vi "Read SCPI Error Queue (GPIB).vi"(2 "error in":T1, 3 "GPIB address":string) -> (0 "error out":T1, 1 "messages":string)   [LabVIEW 2024]
doc: "This VI reads the status message from the power meter and determines whether an error has occurred during the previous operations. If an error is detected, the front panel LED (error) will be turned on, and the messages will be displayed."
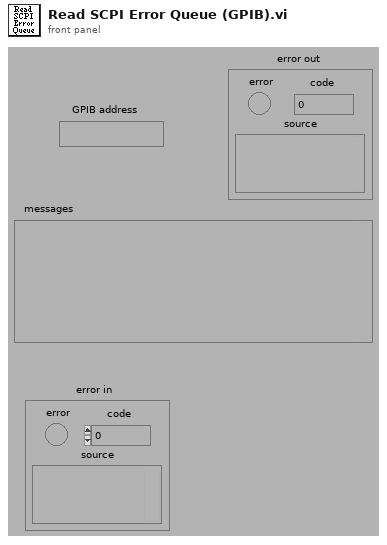
[diagram p1: front panel]
types:
  T1 = cluster{"error":bool, "code":i32, "source":string}
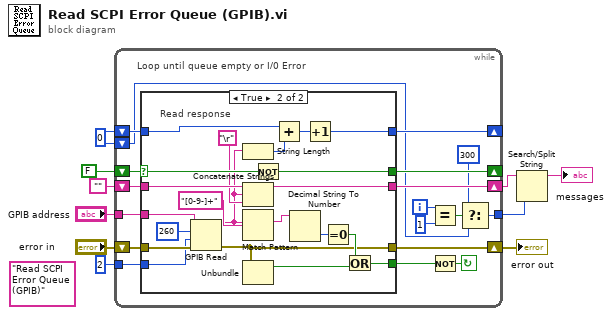
[diagram p0: block diagram]
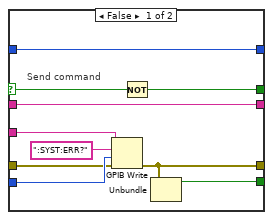
[diagram p2: hidden frame]
diagram:
  w7 = 0
  (unwired) "Read SCPI Error Queue (GPIB)"
  n1 = while {
    shift-right: [w28] -> w6
    shift-left: "" -> [w27]
    shift-right: [w23] -> _
    shift-left: FALSE -> [w24]
    tunnel: "GPIB address" -> [w22]
    shift-right: [w20] -> w1
    shift-left: "error in" -> [w21]
    tunnel: 2 -> [w19]
    shift-right: [w17] -> _
    shift-left: w7 -> [w18]
    shift-left: w7 -> [w16]
    tunnel: [w15] -> w4
    i -> [w14]
    stop <- w25 continue-if-true
    # "Loop until queue empty or I/0 Error"
    n2 = case shown="True" w24 {
      selector: w24 -> [w37 w55]
      tunnel: [w35 w58] -> w26
      tunnel: [w38 w57] -> w28
      tunnel: w27 -> [w38 w56]
      tunnel: [w36 w54] -> w23
      tunnel: w22 -> [w32 w41]
      tunnel: [w33 w43] -> w20
      tunnel: w21 -> [w29 w44]
      tunnel: w19 -> [w30 w40]
      tunnel: w18 -> [w34 w49]
      tunnel: [w34 w47] -> w17
      frame False {
        # "Send command"
        n3 = GPIB Write(0:w32, 1:":SYST:ERR?", 2:w30, 3:w29) -> (6:w33:errorcluster)  [unwired: 1 in, 1 out]
        n4 = Not(x=w37) -> (.not. x?=w36:bool)
        n5 = Unbundle(w33) -> ("status"=w35:bool)  [unwired: 2 out]
      }
      frame True {
        # "Read response"
        n6 = GPIB Read(0:w41, 1:260, 2:w40, 3:w44) -> (5:w42:string, 7:w43:errorcluster)  [unwired: 1 in, 1 out]
        n7 = String Length(string=w42) -> (length=w50:i32)
        n8 = Concatenate Strings(w56, w42, "\r") -> (w57:string)
        n9 = Match Pattern(string=w42, regular expression="[0-9-]+") -> (match substring=w45:string)  [unwired: 1 in, 3 out]
        n10 = Unbundle(w43) -> ("status"=w51:bool)  [unwired: 2 out]
        n11 = Not(x=w55) -> (.not. x?=w54:bool)
        n12 = Add(x=w49, y=w50) -> (x+y=w48:i32)
        n13 = Decimal String To Number(string=w45) -> (number=w59:i32)  [unwired: 2 in, 1 out]
        n14 = Increment(x=w48) -> (x+1=w47:i32)
        n15 = Equal To 0?(x=w59) -> (x = 0?=w53:bool)
        n16 = Or(x=w53, y=w51) -> (x .or. y?=w58:bool)
      }
    }
    n17 = Equal?(x=w14, y=1) -> (x = y?=w12:bool)
    n18 = Not(x=w26) -> (.not. x?=w25:bool)
    n19 = Select(t=300, s=w12, f=w16) -> (s? t:f=w15:i32)
  }
  "error out" <- w1
  n20 = Search/Split String(string=w6, offset (0)=w4) -> (substring before match=→"messages":string)  [unwired: 1 in, 2 out]
